vi "Refresh.vi"(8 "error in (no error)":errorcluster, 11 "OpenHW in":refnum<class "OpenHW.lvclass">) -> (0 "error out":errorcluster, 3 "OpenHW out":refnum<class "OpenHW.lvclass">)   [LabVIEW 2022 SP3, in "open-hw-mon-lv.lvlib" / "OpenHW.lvclass"]
uses:
  OpenHW.lvclass
  OpenHW.lvclass/OpenHW.ctl
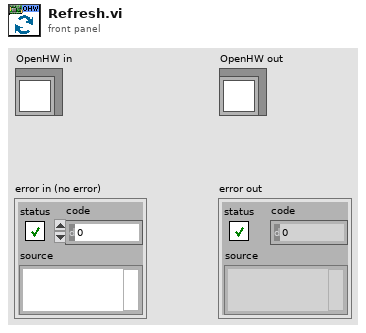
[diagram p1: front panel]
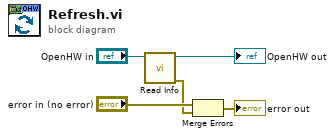
[diagram p0: block diagram]
diagram:
  n1 = call "Read Info.vi"("OpenHW in"="OpenHW in") -> ("error out"=w2:errorcluster, "OpenHW out"=→"OpenHW out":refnum<class "OpenHW.lvclass">)  [unwired: 9 in]
  n2 = Merge Errors("error in (no error)", w2) -> (→"error out":errorcluster)
